vi "Vision.vi"(0 "Image In":T2, 7 "error in":errorcluster) -> (20 "Image Out":T2, 27 "error out":errorcluster)   [LabVIEW 2014]
uses:
  <vilib>/vision/Image Controls.llb/IMAQ Image.ctl
  <vilib>/vision/NI_Vision_Development_Module.lvlib
panel:
  out "Matches out 3":T1(array[cluster])
  out "Results (Calibrated)":sgl[][](array[numeric]) format="%.2f"
  out "Results (Pixels)":sgl[][](array[numeric]) format="%.2f"
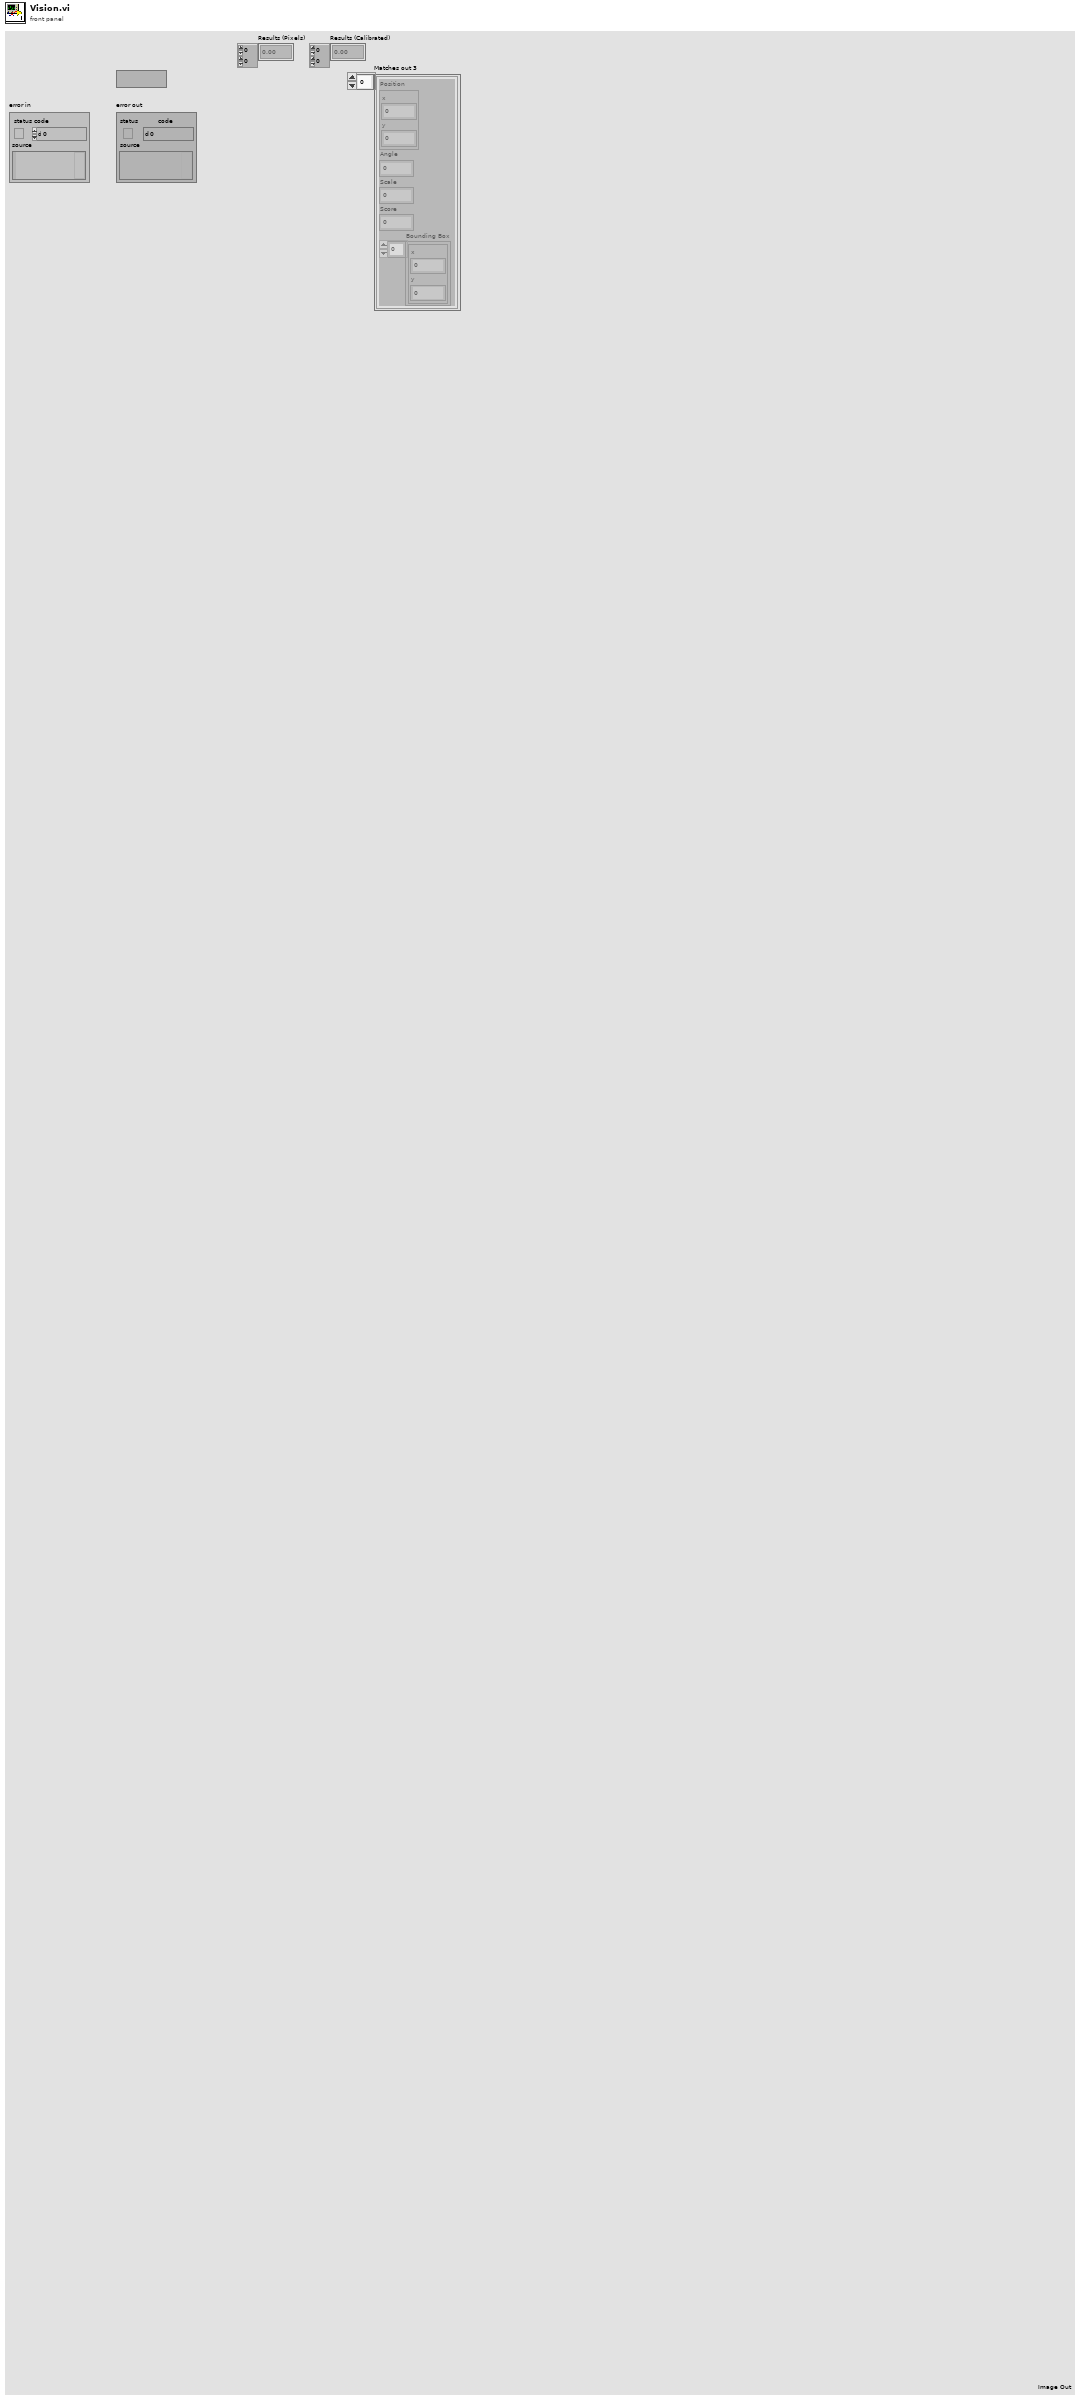
[diagram p1: front panel]
types:
  T1 = cluster{"Position":cluster{"x":sgl, "y":sgl}, "Angle":sgl, "Scale":sgl, "Score":sgl, "Bounding Box":cluster{"x":sgl, "y":sgl}[]}[]
  T2 = typedef "IMAQ Image.ctl" = refnum<image>
  T3 = cluster{"Feature":u32, "Points IDs":cluster{"GUID":string, "Index":i32}[]}[]
  T4 = typedef "Image Type" = u32
  T5 = cluster{"Global Rectangle":i32[], "Contours":cluster{"ID":enum32{"External", "Internal"}, "Type":u32, "Coordinates":i32[]}[]}
  T6 = enum16{"Reset", "Update Coordinate System", "Get Coordinate System"}
  T7 = enum16{"Horizontal Motion", "Vertical Motion", "Horizontal and Vertical Motion", "Horizontal, Vertical and Angular Motion"}
  T8 = cluster{"Origin":cluster{"X":sgl, "Y":sgl}, "Angle (deg)":sgl, "Axis Reference":u32}
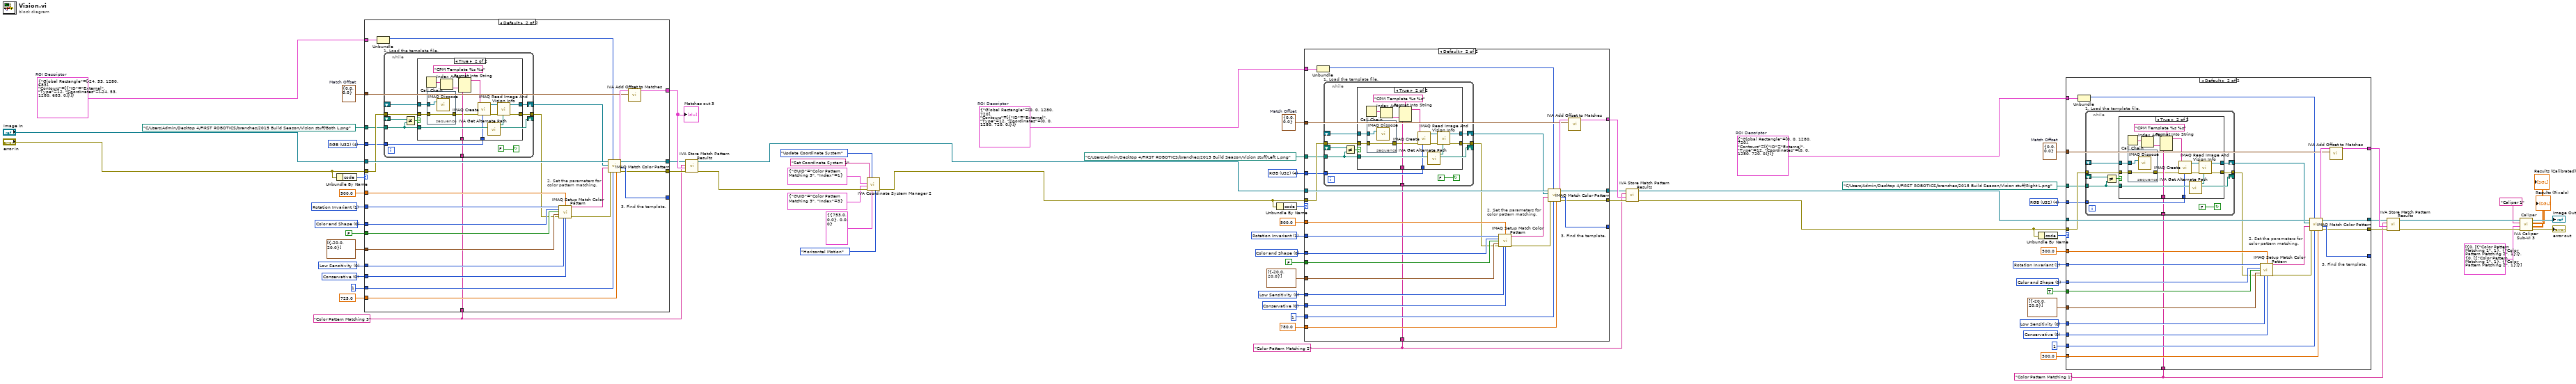
[diagram p0: block diagram]
diagram:
  w8 = "Color Pattern Matching 1" ("Step Name")
  w18 = T4 4 items=["Grayscale (U8)", "Grayscale (I16)", "Grayscale (SGL)", "Complex (CSG)", "RGB (U32)", "HSL (U32)", "RGB (U64)"] ("Image Type")
  w16 = cluster{"X":sgl, "Y":sgl} {"X"=0.0, "Y"=0.0}  # Match Offset
  w21 = u32 0 items=["Conservative", "Balance", "Aggressive", "Very Aggressive"] ("Search Strategy")
  w22 = u32 0 items=["Low Sensitivity", "Medium Sensitivity", "High Sensitivity"] ("Color Sensitivity")
  w24 = u32 0 items=["Color and Shape", "Color", "Shape"] ("Match Feature Mode")
  w25 = u32 1 items=["Shift Invariant", "Rotation Invariant"] ("Match Mode")
  w15 = T5 {"Global Rectangle"=[0, 0, 1280, 720], "Contours"=[{"ID"=enum."External", "Type"=12, "Coordinates"=[0, 0, 1280, 720, 0]}]}  # ROI Descriptor
  w28 = "Color Pattern Matching 2" ("Step Name")
  w38 = T4 4 items=["Grayscale (U8)", "Grayscale (I16)", "Grayscale (SGL)", "Complex (CSG)", "RGB (U32)", "HSL (U32)", "RGB (U64)"] ("Image Type")
  w36 = cluster{"X":sgl, "Y":sgl} {"X"=0.0, "Y"=0.0}  # Match Offset
  w41 = u32 0 items=["Conservative", "Balance", "Aggressive", "Very Aggressive"] ("Search Strategy")
  w42 = u32 0 items=["Low Sensitivity", "Medium Sensitivity", "High Sensitivity"] ("Color Sensitivity")
  w44 = u32 0 items=["Color and Shape", "Color", "Shape"] ("Match Feature Mode")
  w45 = u32 1 items=["Shift Invariant", "Rotation Invariant"] ("Match Mode")
  w35 = T5 {"Global Rectangle"=[0, 0, 1280, 720], "Contours"=[{"ID"=enum."External", "Type"=12, "Coordinates"=[0, 0, 1280, 720, 0]}]}  # ROI Descriptor
  w55 = "Color Pattern Matching 3" ("Step Name")
  w65 = T4 4 items=["Grayscale (U8)", "Grayscale (I16)", "Grayscale (SGL)", "Complex (CSG)", "RGB (U32)", "HSL (U32)", "RGB (U64)"] ("Image Type")
  w63 = cluster{"X":sgl, "Y":sgl} {"X"=0.0, "Y"=0.0}  # Match Offset
  w68 = u32 0 items=["Conservative", "Balance", "Aggressive", "Very Aggressive"] ("Search Strategy")
  w69 = u32 0 items=["Low Sensitivity", "Medium Sensitivity", "High Sensitivity"] ("Color Sensitivity")
  w71 = u32 0 items=["Color and Shape", "Color", "Shape"] ("Match Feature Mode")
  w72 = u32 1 items=["Shift Invariant", "Rotation Invariant"] ("Match Mode")
  w62 = T5 {"Global Rectangle"=[-24, 53, 1280, 683], "Contours"=[{"ID"=enum."External", "Type"=12, "Coordinates"=[-24, 53, 1280, 683, 0]}]}  # ROI Descriptor
  # "Caliper"
  n1 = Unbundle By Name("error in") -> ("code"=w60:i32)
  n2 = case shown="Default" w60 {
    tunnel: 1 ("Number of Matches Requested") -> [_ w101]
    tunnel: sgl 725.0 ("Minimum Match Score") -> [_ w100]
    tunnel: [_ w99] -> _
    tunnel: w72 -> [_ w98]
    tunnel: w71 -> [_ w97]
    tunnel: FALSE ("Subpixel Accuracy") -> [_ w96]
    tunnel: w69 -> [_ w95]
    tunnel: w68 -> [_ w94]
    tunnel: sgl 500.0 ("Color Score Weight") -> [_ w93]
    tunnel: path "C:/Users/Admin/Desktop 4/FIRST ROBOTICS/branches/2015 Build Season/Vision stuff/Both L.png" ("File Path") -> [_ w82]
    tunnel: w65 -> [_ w78]
    tunnel: "error in" -> [_ w83]
    tunnel: cluster{sgl, sgl}[] [{-20.0, 20.0}] ("Rotation Angle Ranges (degrees)") -> [_ w90]
    tunnel: w63 -> [_ w88]
    tunnel: w62 -> [_ w87]
    tunnel: [_ w79] -> w57
    tunnel: "Image In" -> [w76 w84]
    tunnel: [w76 w84] -> w56
    tunnel: [_ w85] -> w59
    tunnel: w55 -> [_ w77]
    frame -1074396199, -1074396198 {
      # "Discard Coordinate System Error"
    }
    frame Default {
      # "2. Set the parameters for\ncolor pattern matching."
      # "3. Find the template."
      n3 = Unbundle(w87) -> ("Global Rectangle"=w86:i32[])  [unwired: 1 out]
      n4 = while "1. Load the template file." {
        shift-right: [w111] -> w81
        shift-left: _ -> [w110]
        tunnel: [w108] -> w80
        tunnel: w83 -> [w107]
        tunnel: w82 -> [w102]
        tunnel: w78 -> [w106]
        tunnel: w77 -> [w105]
        shift-right: [w102] -> _
        shift-left: _ -> [w104]
        stop <- FALSE continue-if-true
        n5 = Not Equal?(x=w104, y=w102) -> (x != y?=w103:bool)
        n6 = case shown="True" w103 {
          tunnel: [w113 w126] -> w111
          tunnel: w110 -> [w113 w118]
          tunnel: [w112 w123] -> w108
          tunnel: w107 -> [w112 w117]
          tunnel: w102 -> [_ w115]
          tunnel: w106 -> [_ w122]
          tunnel: w105 -> [_ w119]
          frame False {
          }
          frame True {
            n7 = Call Chain() -> (call chain=w121:string[])
            n8 = stacked-sequence {
              tunnel: w118 -> [w130]
              tunnel: w117 -> [w129]
              tunnel: [w129] -> w116
              frame #0 {
                n9 = call "IMAQ Dispose"("Image"=w130) -> ()  [unwired: 2 in, 4 out]
              }
            }
            n10 = Index Array(array=w121) -> (element=w120:string)  [unwired: 1 in]
            n11 = Format Into String(format string="CPM Template %s %s" ("Image Name"), w120, w119) -> (resulting string=w128:string)  [unwired: 2 in, 1 out]
            n12 = call "IMAQ Create"("Image Name"=w128, "Image Type"=w122, "error in (no error)"=w116) -> ("New Image"=w125:T2, "error out"=w124:errorcluster)  [unwired: 1 in, 1 out]
            n13 = call <vilib>:"IVA Get Alternate Path.vi"("Path In"=w115) -> ("Path Out"=w114:path)  [unwired: 10 out]
            n14 = call "IMAQ Read Image And Vision Info"("File Path"=w114, "error in (no error)"=w124, "Image"=w125) -> ("error out"=w123:errorcluster, "Image Out"=w126:T2)  [unwired: 1 in, 6 out]
          }
        }
      }
      n15 = call "IMAQ Setup Match Color Pattern"("Match Mode"=w98, "Color Score Weight"=w93, "Match Feature Mode"=w97, "Subpixel Accuracy"=w96, "Rotation Angle Ranges (degrees)"=w90, "error in (no error)"=w80, "Color Sensitivity"=w95, "Search Strategy"=w94) -> ("Match Color Pattern Setup Data"=w92:string, "error out"=w91:errorcluster)  [unwired: 1 in, 5 out]
      n16 = call "IMAQ Match Color Pattern"("Minimum Match Score"=w100, "Number of Matches Requested"=w101, "Optional Rectangle"=w86, "error in (no error)"=w91, "Match Color Pattern Setup Data"=w92, "Template Image"=w81, "Image"=w84) -> ("error out"=w79:errorcluster, "Number of Matches"=w99:i32, "Matches"=w89:T1)  [unwired: 2 out]
      n17 = call <vilib>:"IVA Add Offset to Matches.vi"("Match Offset"=w88, "Matches in"=w89) -> ("Matches out"=w85:T1)  [unwired: 9 out]
    }
  }
  "Matches out 3" <- w59
  n18 = call <vilib>:"IVA Store Match Pattern Results.vi"("error in (no error)"=w57, "Matches"=w59, "Step Name"=w55, "Image in"=w56) -> ("error out"=w58:errorcluster, "Image dup"=w34:T2)  [unwired: 6 out]
  n19 = call <vilib>:"IVA Coordinate System Manager 2.vi"("Mode"=T7."Horizontal Motion", "Reference System"=T8 {"Origin"={"X"=753.0, "Y"=0.0}, "Angle (deg)"=0.0, "Axis Reference"=0}, "Function"=T6."Update Coordinate System", "error in (no error)"=w58, "Angle ID"=cluster{"GUID":string, "Index":i32} {"GUID"="Color Pattern Matching 3", "Index"=3}, "Origin ID"=cluster{"GUID":string, "Index":i32} {"GUID"="Color Pattern Matching 3", "Index"=1}, "Coordinate System Name"="Set Coordinate System 1") -> ("error out"=w48:errorcluster)  [unwired: 4 out]
  n20 = Unbundle By Name(w48) -> ("code"=w33:i32)
  n21 = case shown="Default" w33 {
    tunnel: 1 ("Number of Matches Requested") -> [_ w156]
    tunnel: sgl 780.0 ("Minimum Match Score") -> [_ w155]
    tunnel: [_ w154] -> _
    tunnel: w45 -> [_ w153]
    tunnel: w44 -> [_ w152]
    tunnel: FALSE ("Subpixel Accuracy") -> [_ w151]
    tunnel: w42 -> [_ w150]
    tunnel: w41 -> [_ w149]
    tunnel: sgl 500.0 ("Color Score Weight") -> [_ w148]
    tunnel: path "C:/Users/Admin/Desktop 4/FIRST ROBOTICS/branches/2015 Build Season/Vision stuff/Left L.png" ("File Path") -> [_ w137]
    tunnel: w38 -> [_ w133]
    tunnel: w48 -> [_ w138]
    tunnel: cluster{sgl, sgl}[] [{-20.0, 20.0}] ("Rotation Angle Ranges (degrees)") -> [_ w145]
    tunnel: w36 -> [_ w143]
    tunnel: w35 -> [_ w142]
    tunnel: [_ w134] -> w30
    tunnel: w34 -> [w131 w139]
    tunnel: [w131 w139] -> w29
    tunnel: [_ w140] -> w32
    tunnel: w28 -> [_ w132]
    frame -1074396199, -1074396198 {
      # "Discard Coordinate System Error"
    }
    frame Default {
      # "2. Set the parameters for\ncolor pattern matching."
      # "3. Find the template."
      n22 = Unbundle(w142) -> ("Global Rectangle"=w141:i32[])  [unwired: 1 out]
      n23 = while "1. Load the template file." {
        shift-right: [w166] -> w136
        shift-left: _ -> [w165]
        tunnel: [w163] -> w135
        tunnel: w138 -> [w162]
        tunnel: w137 -> [w157]
        tunnel: w133 -> [w161]
        tunnel: w132 -> [w160]
        shift-right: [w157] -> _
        shift-left: _ -> [w159]
        stop <- FALSE continue-if-true
        n24 = Not Equal?(x=w159, y=w157) -> (x != y?=w158:bool)
        n25 = case shown="True" w158 {
          tunnel: [w168 w181] -> w166
          tunnel: w165 -> [w168 w173]
          tunnel: [w167 w178] -> w163
          tunnel: w162 -> [w167 w172]
          tunnel: w157 -> [_ w170]
          tunnel: w161 -> [_ w177]
          tunnel: w160 -> [_ w174]
          frame False {
          }
          frame True {
            n26 = Call Chain() -> (call chain=w176:string[])
            n27 = stacked-sequence {
              tunnel: w173 -> [w185]
              tunnel: w172 -> [w184]
              tunnel: [w184] -> w171
              frame #0 {
                n28 = call "IMAQ Dispose"("Image"=w185) -> ()  [unwired: 2 in, 4 out]
              }
            }
            n29 = Index Array(array=w176) -> (element=w175:string)  [unwired: 1 in]
            n30 = Format Into String(format string="CPM Template %s %s" ("Image Name"), w175, w174) -> (resulting string=w183:string)  [unwired: 2 in, 1 out]
            n31 = call "IMAQ Create"("Image Name"=w183, "Image Type"=w177, "error in (no error)"=w171) -> ("New Image"=w180:T2, "error out"=w179:errorcluster)  [unwired: 1 in, 1 out]
            n32 = call <vilib>:"IVA Get Alternate Path.vi"("Path In"=w170) -> ("Path Out"=w169:path)  [unwired: 10 out]
            n33 = call "IMAQ Read Image And Vision Info"("File Path"=w169, "error in (no error)"=w179, "Image"=w180) -> ("error out"=w178:errorcluster, "Image Out"=w181:T2)  [unwired: 1 in, 6 out]
          }
        }
      }
      n34 = call "IMAQ Setup Match Color Pattern"("Match Mode"=w153, "Color Score Weight"=w148, "Match Feature Mode"=w152, "Subpixel Accuracy"=w151, "Rotation Angle Ranges (degrees)"=w145, "error in (no error)"=w135, "Color Sensitivity"=w150, "Search Strategy"=w149) -> ("Match Color Pattern Setup Data"=w147:string, "error out"=w146:errorcluster)  [unwired: 1 in, 5 out]
      n35 = call "IMAQ Match Color Pattern"("Minimum Match Score"=w155, "Number of Matches Requested"=w156, "Optional Rectangle"=w141, "error in (no error)"=w146, "Match Color Pattern Setup Data"=w147, "Template Image"=w136, "Image"=w139) -> ("error out"=w134:errorcluster, "Number of Matches"=w154:i32, "Matches"=w144:T1)  [unwired: 2 out]
      n36 = call <vilib>:"IVA Add Offset to Matches.vi"("Match Offset"=w143, "Matches in"=w144) -> ("Matches out"=w140:T1)  [unwired: 9 out]
    }
  }
  n37 = call <vilib>:"IVA Store Match Pattern Results.vi"("error in (no error)"=w30, "Matches"=w32, "Step Name"=w28, "Image in"=w29) -> ("error out"=w31:errorcluster, "Image dup"=w14:T2)  [unwired: 6 out]
  n38 = Unbundle By Name(w31) -> ("code"=w13:i32)
  n39 = case shown="Default" w13 {
    tunnel: 1 ("Number of Matches Requested") -> [_ w211]
    tunnel: sgl 500.0 ("Minimum Match Score") -> [_ w210]
    tunnel: [_ w209] -> _
    tunnel: w25 -> [_ w208]
    tunnel: w24 -> [_ w207]
    tunnel: TRUE ("Subpixel Accuracy") -> [_ w206]
    tunnel: w22 -> [_ w205]
    tunnel: w21 -> [_ w204]
    tunnel: sgl 500.0 ("Color Score Weight") -> [_ w203]
    tunnel: path "C:/Users/Admin/Desktop 4/FIRST ROBOTICS/branches/2015 Build Season/Vision stuff/Right L.png" ("File Path") -> [_ w192]
    tunnel: w18 -> [_ w188]
    tunnel: w31 -> [_ w193]
    tunnel: cluster{sgl, sgl}[] [{-20.0, 20.0}] ("Rotation Angle Ranges (degrees)") -> [_ w200]
    tunnel: w16 -> [_ w198]
    tunnel: w15 -> [_ w197]
    tunnel: [_ w189] -> w10
    tunnel: w14 -> [w186 w194]
    tunnel: [w186 w194] -> w9
    tunnel: [_ w195] -> w12
    tunnel: w8 -> [_ w187]
    frame -1074396199, -1074396198 {
      # "Discard Coordinate System Error"
    }
    frame Default {
      # "2. Set the parameters for\ncolor pattern matching."
      # "3. Find the template."
      n40 = Unbundle(w197) -> ("Global Rectangle"=w196:i32[])  [unwired: 1 out]
      n41 = while "1. Load the template file." {
        shift-right: [w221] -> w191
        shift-left: _ -> [w220]
        tunnel: [w218] -> w190
        tunnel: w193 -> [w217]
        tunnel: w192 -> [w212]
        tunnel: w188 -> [w216]
        tunnel: w187 -> [w215]
        shift-right: [w212] -> _
        shift-left: _ -> [w214]
        stop <- FALSE continue-if-true
        n42 = Not Equal?(x=w214, y=w212) -> (x != y?=w213:bool)
        n43 = case shown="True" w213 {
          tunnel: [w223 w236] -> w221
          tunnel: w220 -> [w223 w228]
          tunnel: [w222 w233] -> w218
          tunnel: w217 -> [w222 w227]
          tunnel: w212 -> [_ w225]
          tunnel: w216 -> [_ w232]
          tunnel: w215 -> [_ w229]
          frame False {
          }
          frame True {
            n44 = Call Chain() -> (call chain=w231:string[])
            n45 = stacked-sequence {
              tunnel: w228 -> [w240]
              tunnel: w227 -> [w239]
              tunnel: [w239] -> w226
              frame #0 {
                n46 = call "IMAQ Dispose"("Image"=w240) -> ()  [unwired: 2 in, 4 out]
              }
            }
            n47 = Index Array(array=w231) -> (element=w230:string)  [unwired: 1 in]
            n48 = Format Into String(format string="CPM Template %s %s" ("Image Name"), w230, w229) -> (resulting string=w238:string)  [unwired: 2 in, 1 out]
            n49 = call "IMAQ Create"("Image Name"=w238, "Image Type"=w232, "error in (no error)"=w226) -> ("New Image"=w235:T2, "error out"=w234:errorcluster)  [unwired: 1 in, 1 out]
            n50 = call <vilib>:"IVA Get Alternate Path.vi"("Path In"=w225) -> ("Path Out"=w224:path)  [unwired: 10 out]
            n51 = call "IMAQ Read Image And Vision Info"("File Path"=w224, "error in (no error)"=w234, "Image"=w235) -> ("error out"=w233:errorcluster, "Image Out"=w236:T2)  [unwired: 1 in, 6 out]
          }
        }
      }
      n52 = call "IMAQ Setup Match Color Pattern"("Match Mode"=w208, "Color Score Weight"=w203, "Match Feature Mode"=w207, "Subpixel Accuracy"=w206, "Rotation Angle Ranges (degrees)"=w200, "error in (no error)"=w190, "Color Sensitivity"=w205, "Search Strategy"=w204) -> ("Match Color Pattern Setup Data"=w202:string, "error out"=w201:errorcluster)  [unwired: 1 in, 5 out]
      n53 = call "IMAQ Match Color Pattern"("Minimum Match Score"=w210, "Number of Matches Requested"=w211, "Optional Rectangle"=w196, "error in (no error)"=w201, "Match Color Pattern Setup Data"=w202, "Template Image"=w191, "Image"=w194) -> ("error out"=w189:errorcluster, "Number of Matches"=w209:i32, "Matches"=w199:T1)  [unwired: 2 out]
      n54 = call <vilib>:"IVA Add Offset to Matches.vi"("Match Offset"=w198, "Matches in"=w199) -> ("Matches out"=w195:T1)  [unwired: 9 out]
    }
  }
  n55 = call <vilib>:"IVA Store Match Pattern Results.vi"("error in (no error)"=w10, "Matches"=w12, "Step Name"=w8, "Image in"=w9) -> ("error out"=w11:errorcluster, "Image dup"=w7:T2)  [unwired: 6 out]
  n56 = call <vilib>:"IVA Caliper Sub-VI 3.vi"("error in"=w11, "Parameters"=T3 [{"Feature"=0, "Points IDs"=[{"GUID"="Color Pattern Matching 1", "Index"=1}, {"GUID"="Color Pattern Matching 2", "Index"=1}]}, {"Feature"=0, "Points IDs"=[{"GUID"="Color Pattern Matching 1", "Index"=1}, {"GUID"="Color Pattern Matching 2", "Index"=1}]}], "Step Name"="Caliper 1", "Image In"=w7) -> ("error out"=→"error out":errorcluster, "Results (Calibrated)"=→"Results (Calibrated)":sgl[][], "Results (Pixels)"=→"Results (Pixels)":sgl[][], "Image Out"=→"Image Out":T2)  [unwired: 1 in, 3 out]
